vi "kalman predict step single cycle.vi"(7 "v-feedback":bool, 10 "state in":T1) -> (2 "state out":T1)   [LabVIEW 2010]
uses:
  integrating single axis kalman state.ctl
  <vilib>/rvi/FXPMathLib/FxpAdd/XNode/nifxpmath_Add.xnode
  <vilib>/rvi/FXPMathLib/FxpAdd/subVIs/nifxpmath_Add_SimConfig.ctl
  <vilib>/fxp/LVFixedPointQuantizationPolicyTypeDef.ctl
  <vilib>/fxp/LVFixedPointOverflowPolicyTypeDef.ctl
  <vilib>/rvi/FXPMathLib/FxpInterpret/XNode/nifxpmath_Interpret.xnode
  <vilib>/rvi/FXPMathLib/FxpAdd/simVIs/DllFxpAddTemp_sub.vi
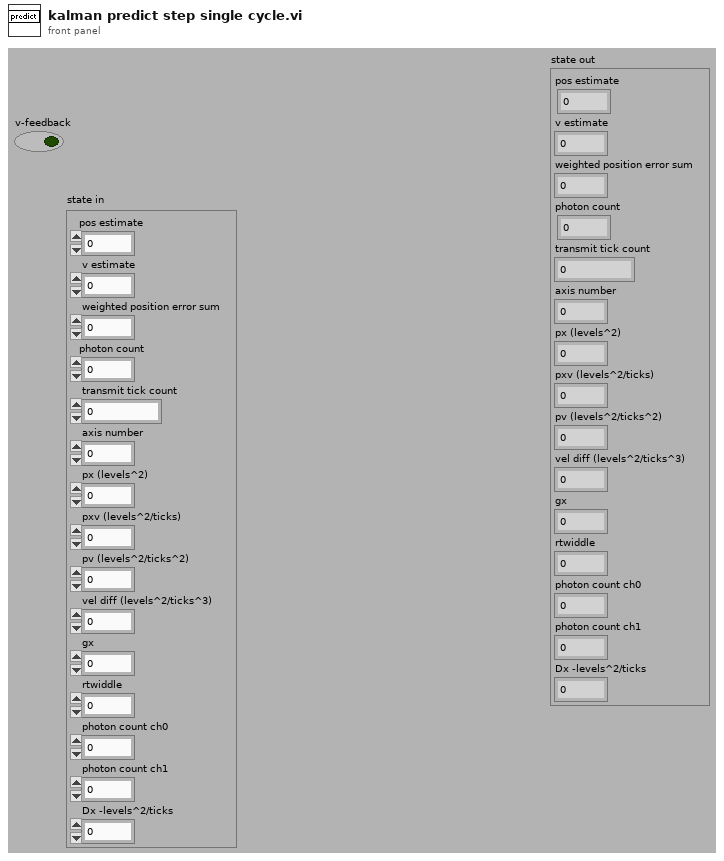
[diagram p1: front panel]
types:
  T1 = typedef "integrating single axis kalman state.ctl" = cluster{"pos estimate":fxp<+/-,32,16>, "v estimate":fxp<+/-,16,0>, "weighted position error sum":fxp<+/-,32,32>, "photon count":u32, "transmit tick count":u32, "axis number":u8, "px (levels^2)":fxp<+,32,19>, "pxv (levels^2/ticks)":fxp<+,32,2>, "pv (levels^2/ticks^2)":fxp<+,32,-14>, "vel diff (levels^2/ticks^3)":fxp<+,24,-22>, "gx":fxp<+,16,8>, "rtwiddle":fxp<+,16,26>, "photon count ch0":u32, "photon count ch1":u32, "Dx -levels^2/ticks":fxp<+,32,19>}
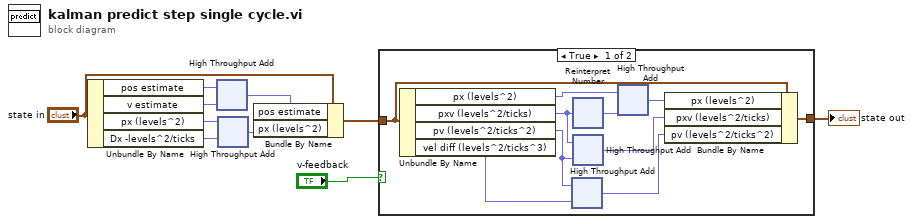
[diagram p0: block diagram]
diagram:
  n1 = Unbundle By Name("state in") -> ("pos estimate"=w5:fxp<+/-,32,16>, "v estimate"=w8:fxp<+/-,16,0>, "px (levels^2)"=w7:fxp<+,32,19>, "Dx -levels^2/ticks"=w3:fxp<+,32,19>)
  n2 = xnode "High Throughput Add"("x"=w5, "y"=w8) -> ("x+y"=w4:fxp<+/-,32,16>)
  n3 = xnode "High Throughput Add"("x"=w7, "y"=w3) -> ("x+y"=w6:fxp<+,32,19>)
  n4 = Bundle By Name(cluster="state in", "pos estimate"=w4, "px (levels^2)"=w6) -> (w1:T1)
  n5 = case shown="True" "v-feedback" {
    tunnel: w1 -> [w15 w116]
    tunnel: [w11 w116] -> w10
    frame True {
      n6 = Unbundle By Name(w15) -> ("px (levels^2)"=w20:fxp<+,32,19>, "pxv (levels^2/ticks)"=w18:fxp<+,32,2>, "pv (levels^2/ticks^2)"=w17:fxp<+,32,-14>, "vel diff (levels^2/ticks^3)"=w16:fxp<+,24,-22>)
      n7 = xnode "High Throughput Add"("x"=w17, "y"=w16) -> ("x+y"=w12:fxp<+,32,-14>)
      n8 = xnode "Reinterpret Number"("x"=w18) -> ("y"=w19:fxp<+,32,3>)
      n9 = xnode "High Throughput Add"("x"=w18, "y"=w17) -> ("x+y"=w13:fxp<+,32,2>)
      n10 = xnode "High Throughput Add"("x"=w20, "y"=w19) -> ("x+y"=w14:fxp<+,32,19>)
      n11 = Bundle By Name(cluster=w15, "px (levels^2)"=w14, "pxv (levels^2/ticks)"=w13, "pv (levels^2/ticks^2)"=w12) -> (w11:T1)
    }
    frame False {
    }
  }
  "state out" <- w10
